vi "IBM4_Close.vi"(8 "error in":errorcluster, 11 "COM resource in":refnum<visa-resource-name>="COM3") -> (0 "error out":errorcluster)   [LabVIEW 2021, in "IBM4.lvlib"]
doc: "This VI is used to close the IBM4. This should always be the last sub-VI called. If it is neglected, your computer may run out of resources, and eventually you will not be able to connect to the IBM4. This can sometimes be rectifies by calling this VI repeatedly. Otherwise, you may need to reboot your computer.\n\nFor proper operation, the input Com port must be one that has previously been opened by the sub-VI IBM4_Open."
uses:
  <instrlib>/IBM4/IBM4.lvlib
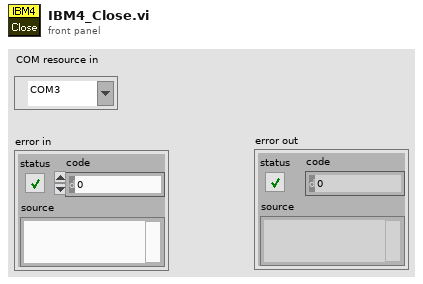
[diagram p1: front panel]
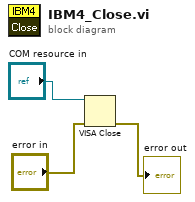
[diagram p0: block diagram]
diagram:
  n1 = VISA Close(VISA resource name="COM resource in", error in (no error)="error in") -> (error out=→"error out":errorcluster)
